vi "Raster_2DOutput_wCounter_82.vi"() -> ()   [LabVIEW 2011]
uses:
  <vilib>/DAQmx/write.llb/DAQmx Write (Analog 2D DBL NChan NSamp).vi
  <vilib>/DAQmx/read.llb/DAQmx Read (Counter 1D U32 1Chan NSamp).vi
  <vilib>/DAQmx/create/channels.llb/DAQmx Create Channel (CI-Period).vi
  <vilib>/DAQmx/create/channels.llb/DAQmx Create Channel (AO-Voltage-Basic).vi
  <vilib>/DAQmx/configure/timing.llb/DAQmx Timing (Implicit).vi
  <vilib>/DAQmx/configure/timing.llb/DAQmx Timing (Sample Clock).vi
  <vilib>/DAQmx/miscellaneous.llb/DAQmx Fill In Error Info.vi
  Program Files/National Instruments/LabVIEW 2011/resource/objmgr/daqmx.rc
panel:
  in  "Save?":bool
  in  "Save File path":path
  out "TotalSampPerChanAcquired":dbl
  out "Spectrogram:":dbl[][](graph)
  out "Output:":dbl[][](graph)
  in  "Y Parameters":T1
  in  "X Parameters":T2
  in  "stop":bool
  in  "Update Rate (Hz)":dbl=100000.0
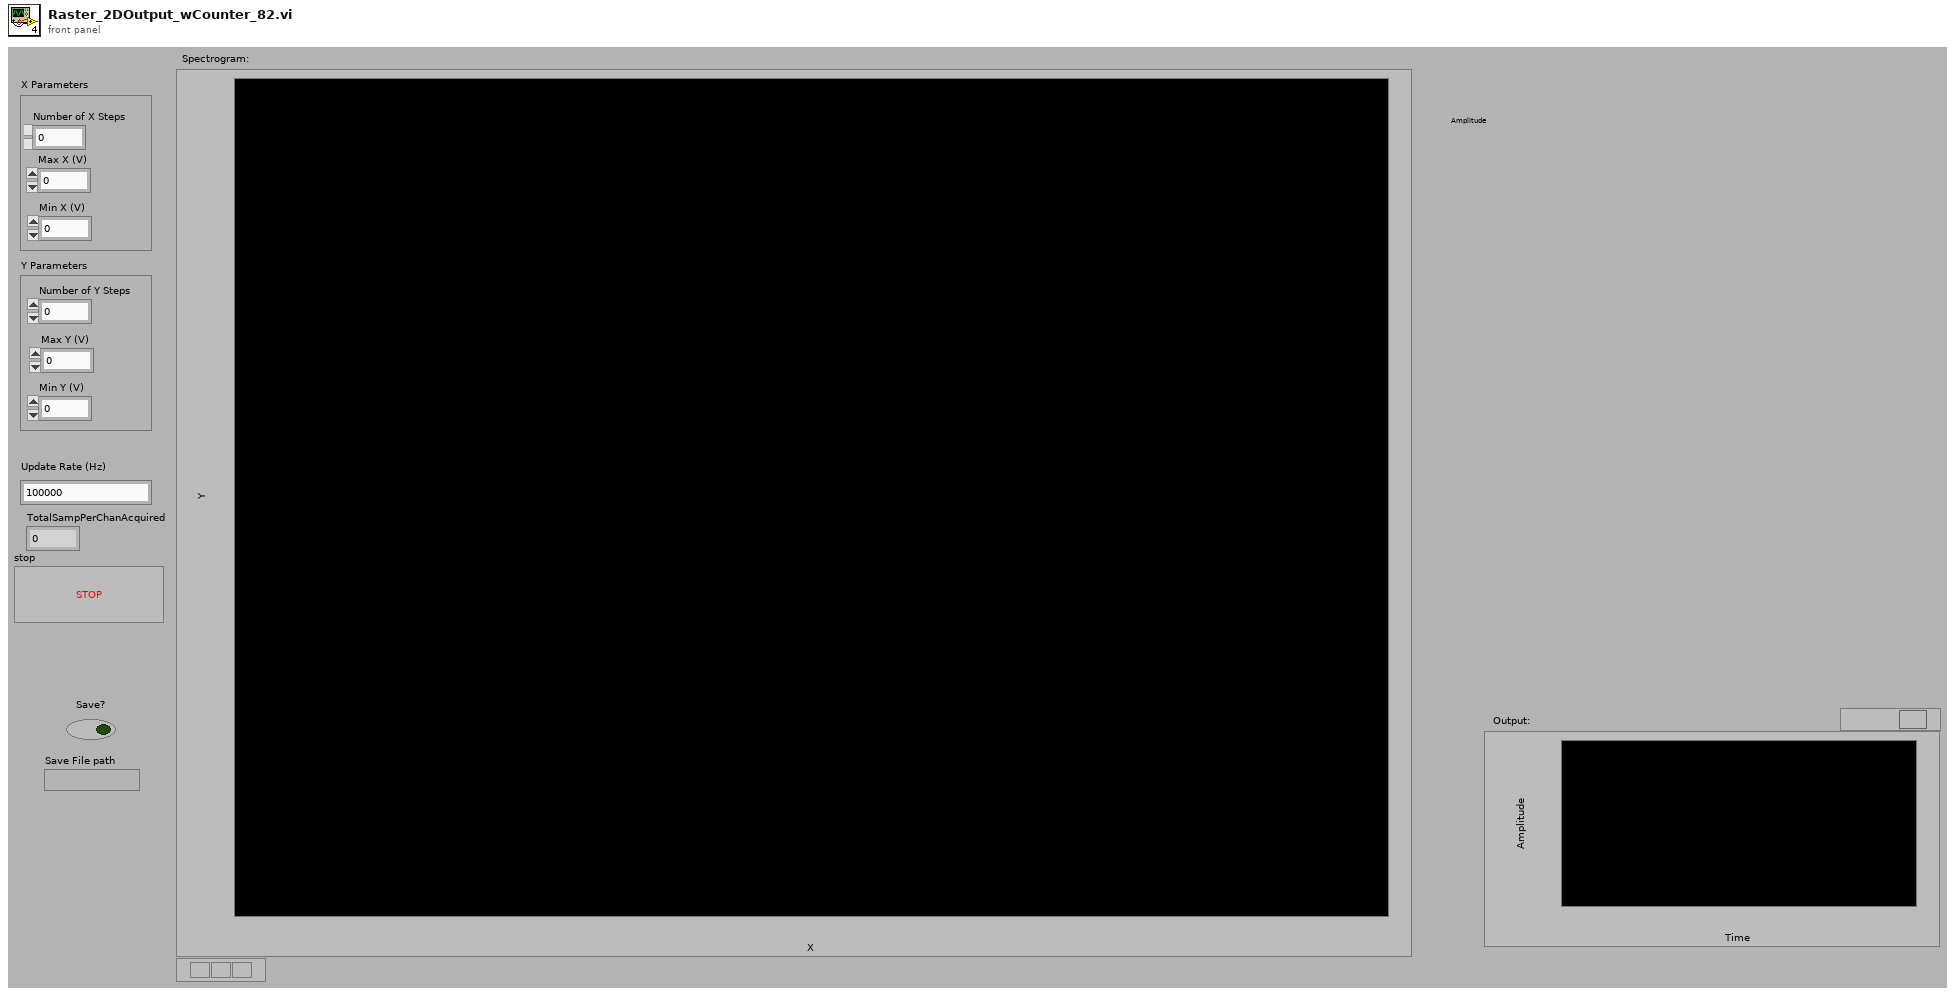
[diagram p1: front panel]
types:
  T1 = cluster{"Number of Y Steps":i32, "Max Y (V)":dbl, "Min Y (V)":dbl}
  T2 = cluster{"Number of X Steps":i32, "Max X (V)":dbl, "Min X (V)":dbl}
  T3 = typedef "imagedata.ctl" = cluster{"image type":i32, "image depth":i32, "image":u8[], "mask":u8[], "colors":u32[], "Rectangle":cluster{"left":i16, "top":i16, "right":i16, "bottom":i16}}
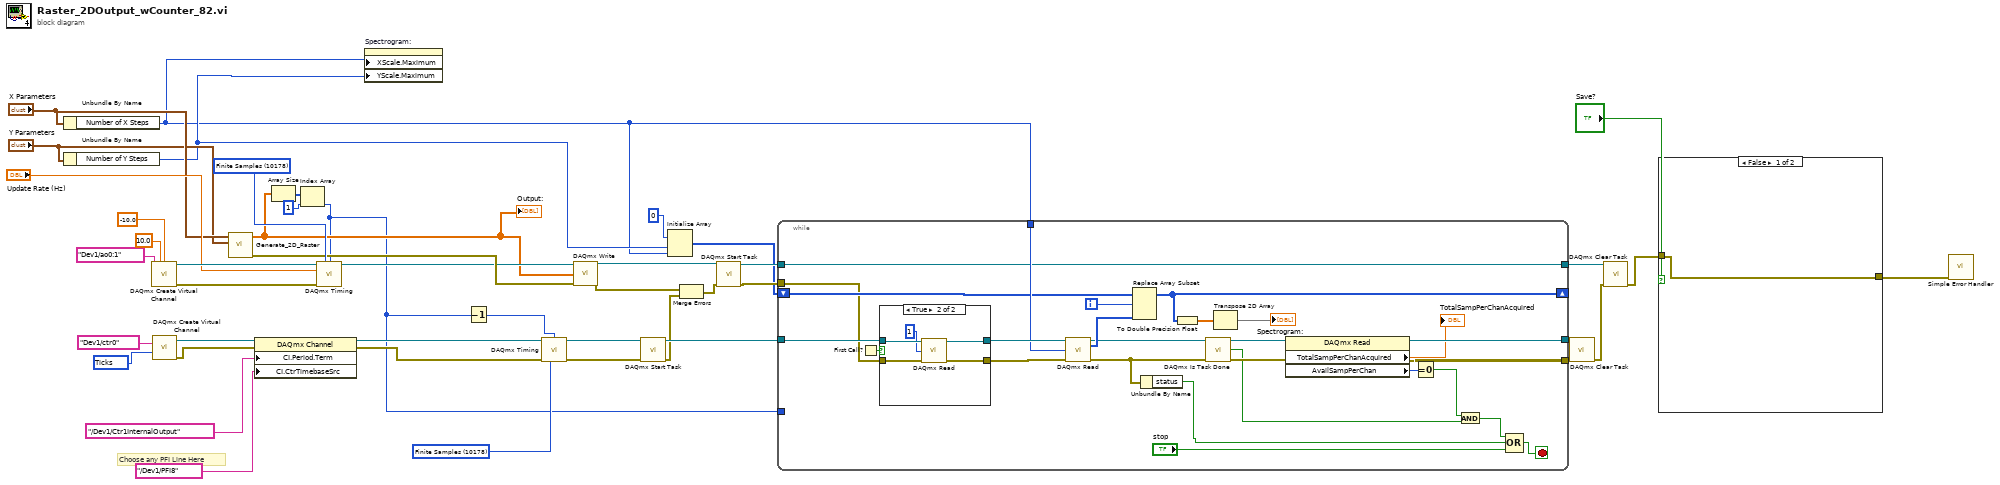
[diagram p0: block diagram]
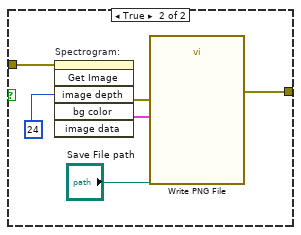
[diagram p2: hidden frame]
diagram:
  w27 = 10178 items=["Finite Samples"=10178, "Continuous Samples"=10123, "Hardware Timed Single Point"=12522] ("sample mode")
  w28 = 10178 items=["Finite Samples"=10178, "Continuous Samples"=10123, "Hardware Timed Single Point"=12522] ("sample mode")
  w41 = 10304 items=["Seconds"=10364, "Ticks"=10304, "From Custom Scale"=10065] ("units")
  # "Choose any PFI Line Here"
  n1 = Unbundle By Name("X Parameters") -> ("Number of X Steps"=w8:i32)
  n2 = Unbundle By Name("Y Parameters") -> ("Number of Y Steps"=w9:i32)
  n3 = call-poly <vilib>:"DAQmx Create Virtual Channel.vi"("maximum value"=10.0, "minimum value"=-10.0, "physical channels"=tag "Dev1/ao0:1") -> ("task out"=w45:refnum<k21>, "error out"=w44:errorcluster)  [unwired: 6 in, 5 out]
  n4 = call-poly <vilib>:"DAQmx Create Virtual Channel.vi"("counter"=tag "Dev1/ctr0", "units"=w41) -> ("task out"=w40:refnum<k21>, "error out"=w39:errorcluster)  [unwired: 10 in, 2 out]
  n5 = call "Generate_2D_Raster.vi"("Y Parameters"="Y Parameters", "X Parameters"="X Parameters") -> ("error IO"=w18:errorcluster, "Array"=w12:dbl[][])  [unwired: 1 in, 7 out]
  "Output:" <- w12
  n6 = property class="DAQmx Channel"(reference=w40, error in=w39, "CI.Period.Term"=tag "/Dev1/Ctr1InternalOutput", "CI.CtrTimebaseSrc"=tag "/Dev1/PFI8") -> (reference out=w38:refnum<k21>, error out=w37:errorcluster)
  n7 = Array Size(array=w12) -> (size(s)=w11:i32[])
  n8 = Index Array(array=w11, index=1) -> (element=w7:i32)
  n9 = call-poly <vilib>:"DAQmx Timing.vi"("task/channels in"=w45, "sample mode"=w28, "samples per channel"=w7, "rate"="Update Rate (Hz)", "error in"=w44) -> ("task out"=w13:refnum<k21>)  [unwired: 2 in, 8 out]
  n10 = property on="Spectrogram:" class="IntGraph (strict)"("XScale.Maximum"=w8, "YScale.Maximum"=w9) -> ()  [unwired: 2 in, 2 out]
  n11 = Decrement(x=w7) -> (x-1=w4:i32)
  n12 = call-poly <vilib>:"DAQmx Timing.vi"("task/channels in"=w38, "sample mode"=w27, "samples per channel"=w4, "error in"=w37) -> ("task out"=w34:refnum<k21>, "error out"=w33:errorcluster)  [unwired: 10 out]
  n13 = call-poly <vilib>:"DAQmx Write.vi"("task/channels in"=w13, "data"=w12, "error in"=w18) -> ("task out"=w32:refnum<k21>, "error out"=w20:errorcluster)  [unwired: 1 in, 10 out]
  n14 = call <vilib>:"DAQmx Start Task.vi"("task/channels in"=w34, "error in"=w33) -> ("task out"=w29:refnum<k21>, "error out"=w19:errorcluster)  [unwired: 12 out]
  n15 = Initialize Array(u32 0, w9, w8) -> (w14:u32[][])
  n16 = Merge Errors(w20, w19) -> (w21:errorcluster)
  n17 = call <vilib>:"DAQmx Start Task.vi"("task/channels in"=w32, "error in"=w21) -> ("task out"=w30:refnum<k21>, "error out"=w31:errorcluster)  [unwired: 12 out]
  n18 = while {
    tunnel: w30 -> [w61]
    tunnel: w31 -> [w62]
    tunnel: w29 -> [w70]
    tunnel: [w61] -> w26
    tunnel: w8 -> [w66]
    shift-right: [w63] -> _
    shift-left: w14 -> [w65]
    tunnel: w7 -> [_]
    tunnel: [w55] -> w6
    tunnel: [w56] -> w5
    i -> [w64]
    stop <- w71 stop-if-true
    n19 = First Call?() -> (First Call?: T/F=w67:bool)
    n20 = case shown="True" w67 {
      tunnel: w70 -> [w74 w79]
      tunnel: [w74 w78] -> w69
      tunnel: [w73 w77] -> w68
      tunnel: w62 -> [w73 w76]
      frame False {
      }
      frame True {
        n21 = call-poly <vilib>:"DAQmx Read.vi"("task/channels in"=w79, "number of samples per channel"=1, "error in"=w76) -> ("task out"=w78:refnum<k21>, "error out"=w77:errorcluster)  [unwired: 11 out]
      }
    }
    n22 = call-poly <vilib>:"DAQmx Read.vi"("task/channels in"=w69, "number of samples per channel"=w66, "error in"=w68) -> ("task out"=w57:refnum<k21>, "data"=w60:u32[], "error out"=w47:errorcluster)  [unwired: 1 in, 9 out]
    n23 = Replace Array Subset(array=w65, new element=w60, index (row)=w64) -> (w63:u32[][])  [unwired: 1 in]
    n24 = Unbundle By Name(w47) -> ("status"=w46:bool)
    n25 = To Double Precision Float(number=w63) -> (double precision float=w58:dbl[][])
    n26 = call <vilib>:"DAQmx Is Task Done.vi"("task/channels in"=w57, "error in"=w47) -> ("task out"=w54:refnum<k21>, "task done?"=w51:bool, "error out"=w53:errorcluster)  [unwired: 11 out]
    n27 = Transpose 2D Array(2D array=w58) -> (transposed array=→"Spectrogram:":dbl[][])
    n28 = property class="DAQmx Read"(reference=w54, error in=w53) -> (reference out=w56:refnum<k21>, error out=w55:errorcluster, "TotalSampPerChanAcquired"=→"TotalSampPerChanAcquired":dbl, "AvailSampPerChan"=w50:u32)
    n29 = Equal To 0?(x=w50) -> (x = 0?=w49:bool)
    n30 = And(x=w49, y=w51) -> (x .and. y?=w48:bool)
    n31 = Compound Arithmetic op=OR(w48, w46, "stop") -> (w71:bool)
  }
  n32 = call <vilib>:"DAQmx Clear Task.vi"("task in"=w5, "error in"=w6) -> ("error out"=w22:errorcluster)  [unwired: 13 out]
  n33 = call <vilib>:"DAQmx Clear Task.vi"("task in"=w26, "error in"=w22) -> ("error out"=w3:errorcluster)  [unwired: 13 out]
  n34 = case shown="False" "Save?" {
    tunnel: w3 -> [w80 w86]
    tunnel: [w80 w82] -> w2
    frame False {
    }
    frame True {
      n35 = invoke on="Spectrogram:" class="IntGraph (strict)" method="Get Image"(error in=w86, "image depth"=24 ("Image Depth")) -> (error out=w83:errorcluster, "image data"=w84:T3)  [unwired: 4 in, 4 out]
      n36 = call <vilib>:"Write PNG File.vi"("error in (no error)"=w83, "image data"=w84, "path to PNG file"="Save File path") -> ("error out"=w82:errorcluster)  [unwired: 7 in, 1 out]
    }
  }
  n37 = call <vilib>:"Simple Error Handler.vi"("error in (no error)"=w2) -> ()  [unwired: 1 in, 8 out]
